vi "_Persist New Entity.vi"(8 "error in (no error)":errorcluster, 10 "New Entity":refnum<class "Entity.lvclass">, 11 "Entity Manager in":refnum<class "Entity Manager.lvclass">) -> (0 "error out":errorcluster, 2 "Entity ID":T1, 3 "Entity Manager out":refnum<class "Entity Manager.lvclass">)   [LabVIEW 2020, in "Conditum.lvlib" / "Entity Manager.lvclass"]
uses:
  Entity Manager.lvclass
  Database Platform/Database Platform.lvclass
  Entity/Entity.lvclass
  Entity ID.ctl
  Conditum.lvlib
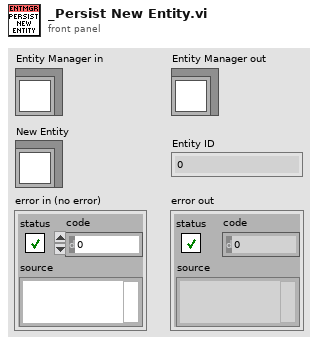
[diagram p1: front panel]
types:
  T1 = typedef "Conditum.lvlib/Entity ID.ctl" = i64
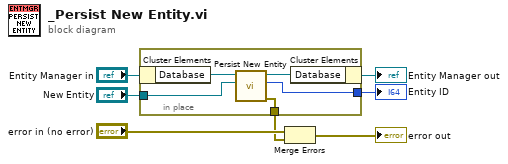
[diagram p0: block diagram]
diagram:
  n1 = in-place {
    in-place-border: "New Entity" -> [w10]
    in-place-border: [w9] -> w4
    in-place-border: [w8] -> w1
    n2 = in-place-cluster #1("Entity Manager in") -> ("Database"=w12:refnum<class "Database Platform.lvclass">)
    n3 = call-dynamic "Persist New Entity.vi"("Entity"=w10, "Database in"=w12) -> ("error out"=w8:errorcluster, "Entity ID"=w9:T1, "Database out"=w11:refnum<class "Database Platform.lvclass">)  [unwired: 7 in]
    n4 = in-place-cluster #1("Database"=w11) -> (→"Entity Manager out":refnum<class "Entity Manager.lvclass">)
  }
  "Entity ID" <- w4
  n5 = Merge Errors("error in (no error)", w1) -> (→"error out":errorcluster)
